vi "RT_BF_LD-400_MFLI_PK_v4.0_measure_voltageR_fourMFLI.vi"() -> ()   [LabVIEW 2016]
uses:
  <instrlib>/Zurich Instruments LabOne/Public/Configure/ziGetValueDemodSampleEx.vi
  <vilib>/Utility/file.llb/Write To Spreadsheet File (DBL).vi
  Labview Drivers/lake_shore_372/Lake Shore 372/Lake Shore 372.lvlib
  <instrlib>/Zurich Instruments LabOne/Zurich Instruments LabOne.lvlib
panel:
  in  "Number average":i32=50
  in  "Current 4 (A)":dbl=1e-09
  in  "Current 3 (A)":dbl=1e-06
  in  "Current 2 (A)":dbl=2e-06
  in  "Current 1 (A)":dbl=2e-06
  in  "MFLI 4 Address":string="DEV3637"
  in  "Device 4 details:":string="VOM133_27.777777Hz_1nA"
  in  "Delay(s) after each data point":dbl format="%#_13g"
  in  "Device 3 details:":string="VOM136_37.7777777Hz_1uA"
  in  "MFLI 3 Address":string="DEV3647"
  in  "MFLI 2 Address":string="DEV4496"
  in  "MFLI 1 Address":string="DEV4382"
  in  "Device 2 details:":string="VOM111_7.919Hz_2uA"
  in  "Device 1 details:":string="VOM134_17.77777Hz_2uA"
  in  "STOP":bool
  out "Device details":string="Device details: \rDevice 1 details: VOM134_17.77777Hz_2uA\tDevice 2 details: VOM111_7.919Hz_2uA\tDevice 3 details: VOM136_37.7777777Hz_1uA\tDevice 4 details: VOM133_27.777777Hz_1nA\t\r"
  out "data":ext[](array[numeric])=[0.0080852, 9923.583, 0.16276936015514457, 1.6064700025522405e-08, 9.869609372556507e-08, 0.27307549143227666, 2.7272832558602143e-08, 9.987286817852663e-08]
  out "path":path=path "D:/Mostafa/17-06-2021/001_RT_cooldown"
  in  "Path":path=path "D:/Mostafa/17-06-2021/001_RT_cooldown"
  in  "Tab Control":enum32{"Page 1", "Page 2"}(tab)
  out "Resistance vs time":cluster{dbl[], dbl[]}[](graph)
  out "Resistance 1 (ohm)":dbl=0.16276936015514457 format="%#_13g"
  out "Voltage 1 (V)":dbl=1.6064700025522405e-08 format="%#_4g"
  out "elapsed time (min)":dbl=165.39305000000002
  out "elapsed time (s)":dbl=9923.583
  out "T MXC (K)":dbl=0.0080852
  out "Resistance vs T":cluster{dbl[], dbl[]}[](graph)
  out "Voltage 2 (V)":dbl=2.7272832558602143e-08 format="%#_4g"
  out "Resistance 2 (ohm)":dbl=0.27307549143227666 format="%#_13g"
  out "Resistance 3 (ohm)":dbl format="%#_13g"
  out "Voltage 3 (V)":dbl=2.7272832558602143e-08 format="%#_4g"
  out "Resistance 4 (ohm)":dbl=0.16276936015514457 format="%#_13g"
  out "Voltage 4 (V)":dbl=2.7272832558602143e-08 format="%#_4g"
  out "Updates":string="- Using shift register to get data from MFLI\n- Using read demod instead of poll function\n- Measuring 2 devices using MFLI at the same time"
  out "Error Out":errorcluster
  # "Use this button to abort the measurement"
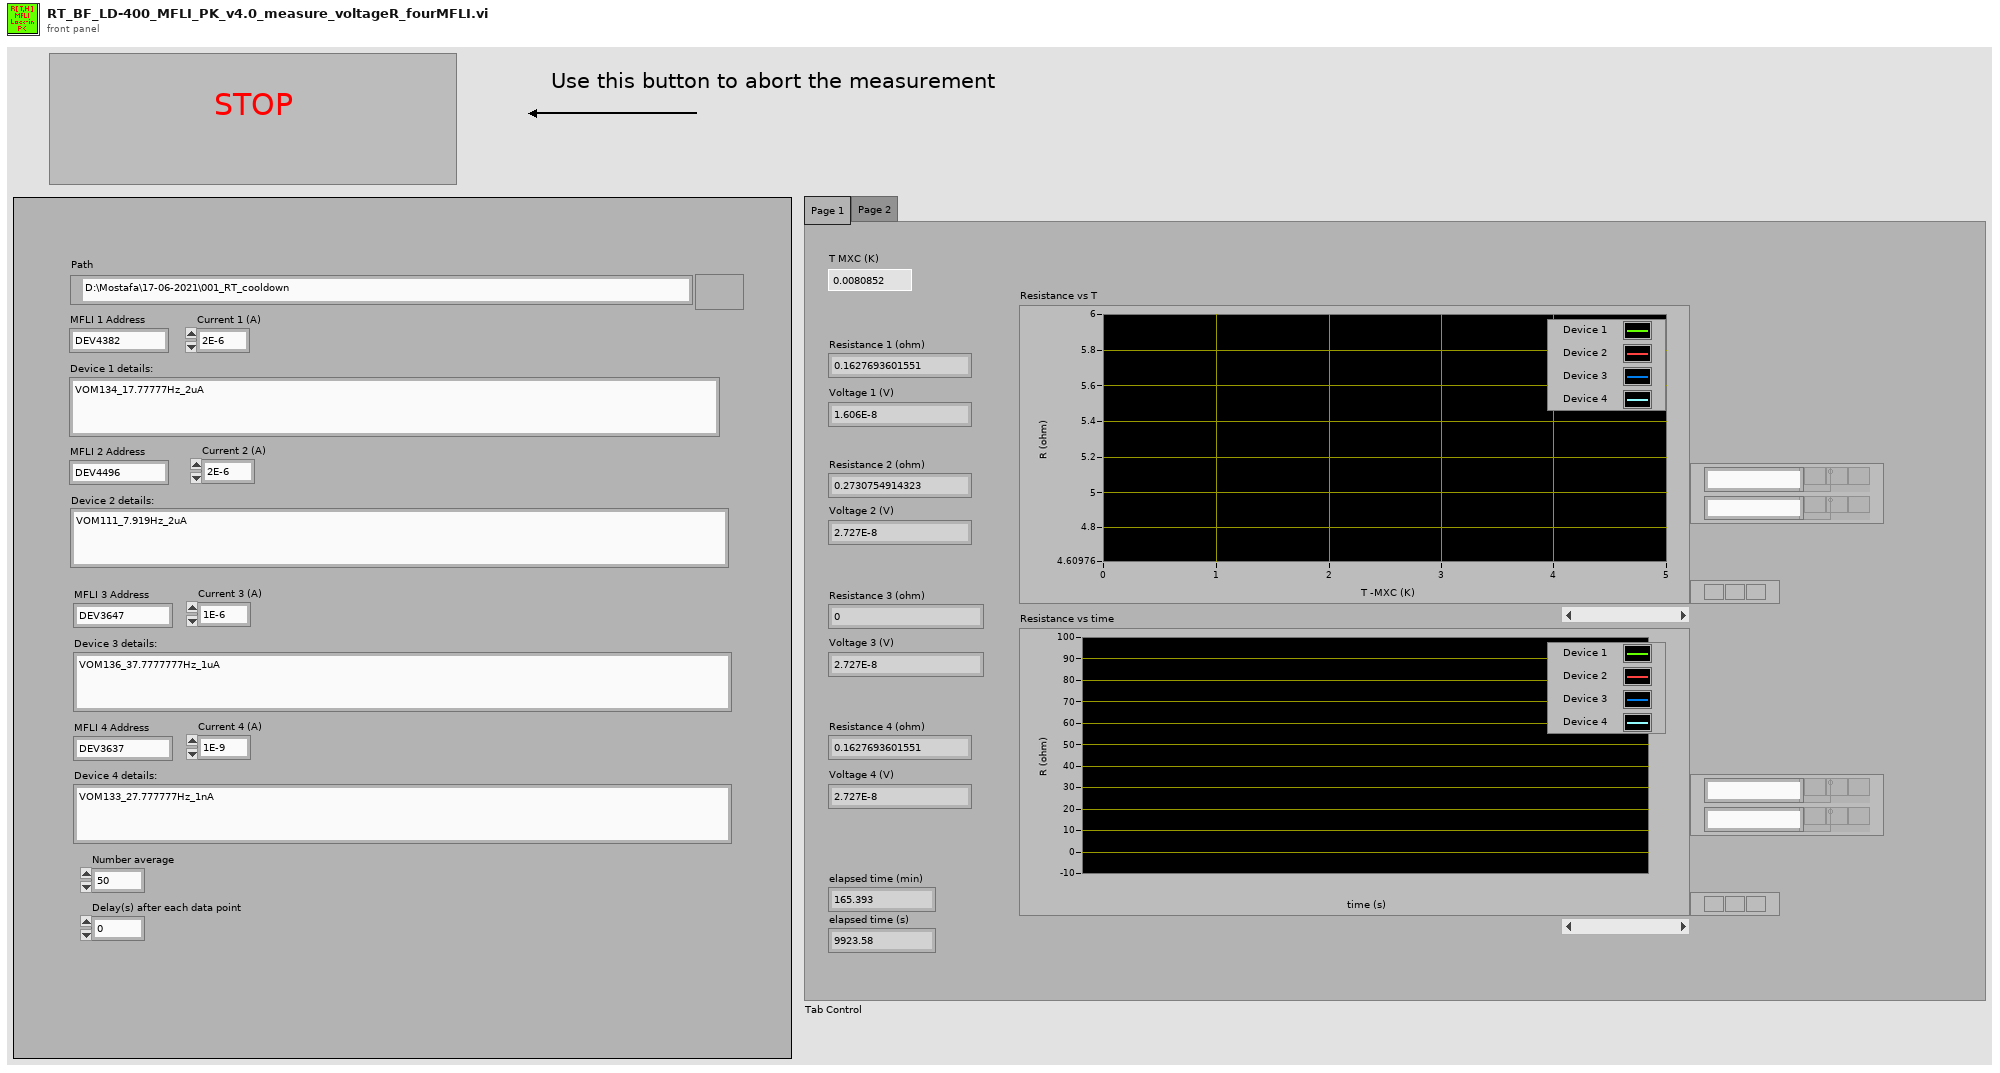
[diagram p1: front panel]
types:
  T1 = enum16{"open", "replace", "create", "open or create", "replace or create", "replace or create with confirmation"}
  T2 = typedef "Zurich Instruments LabOne.lvlib/ziTypeHandle.ctl" = cluster{"handleValid":bool, "Conn":u64, "Path Prefix":string, "Handle":u64, "Connected":bool, "Clockbase(s)":dbl}
  T3 = typedef "Zurich Instruments LabOne.lvlib/ziTypeDemodSampleSingle.ctl" = cluster{"Timestamps (ticks)":u64, "X (Vrms)":dbl, "Y (Vrms)":dbl, "Osc Phase (deg)":dbl, "Freq (Hz)":dbl, "DIO":u32, "AuxIn0 (V)":dbl, "AuxIn1 (V)":dbl, "Trigger":u32}
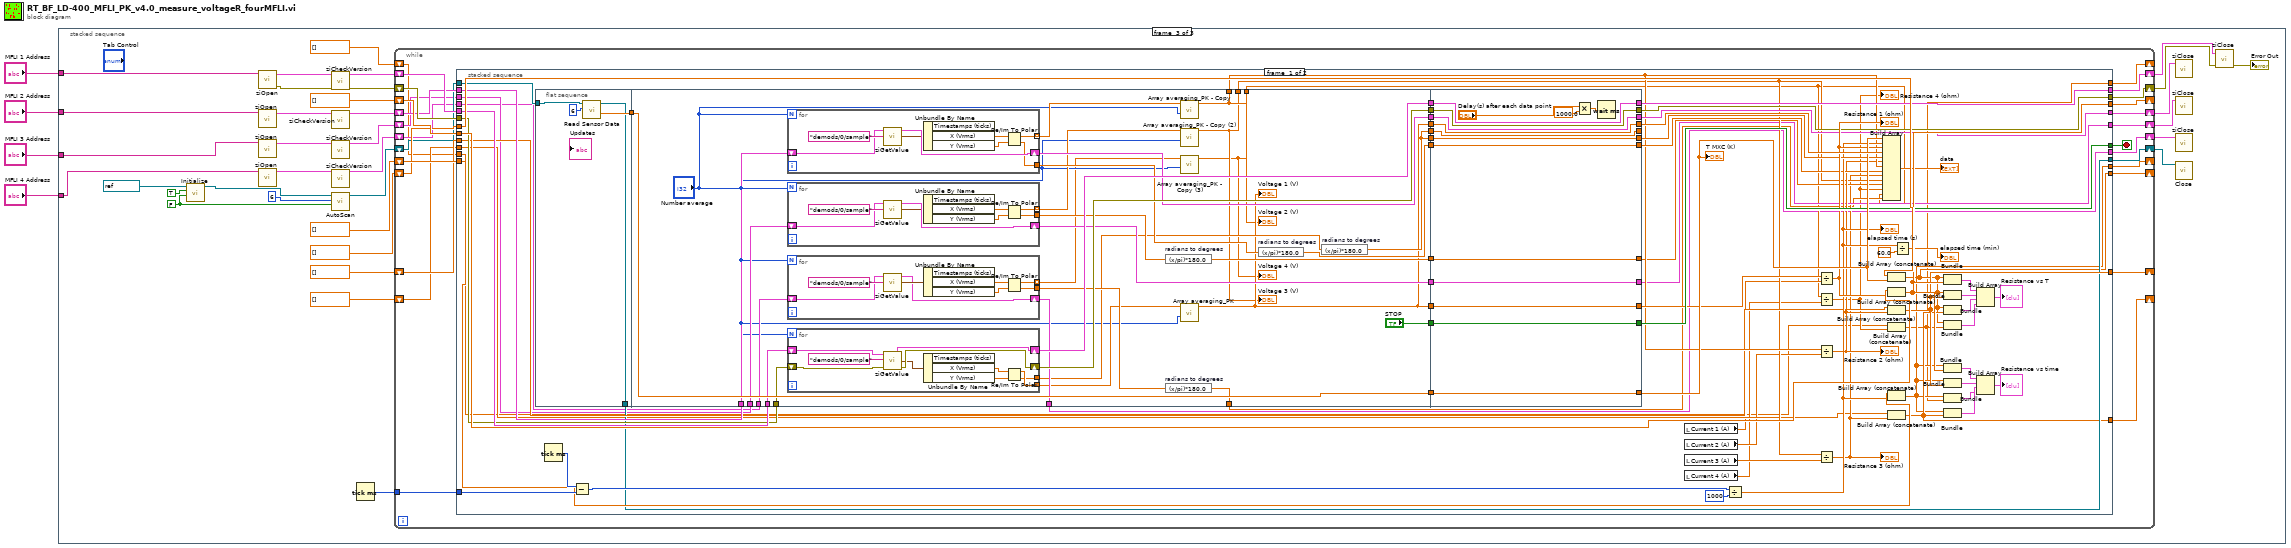
[diagram p0: block diagram]
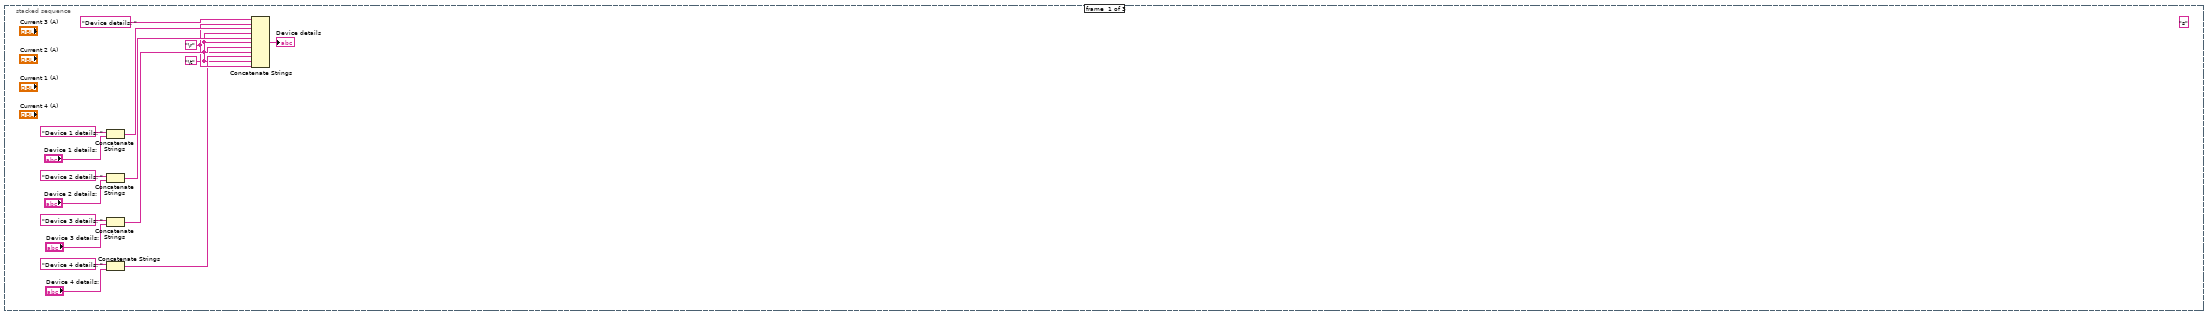
[diagram p2: hidden frame]
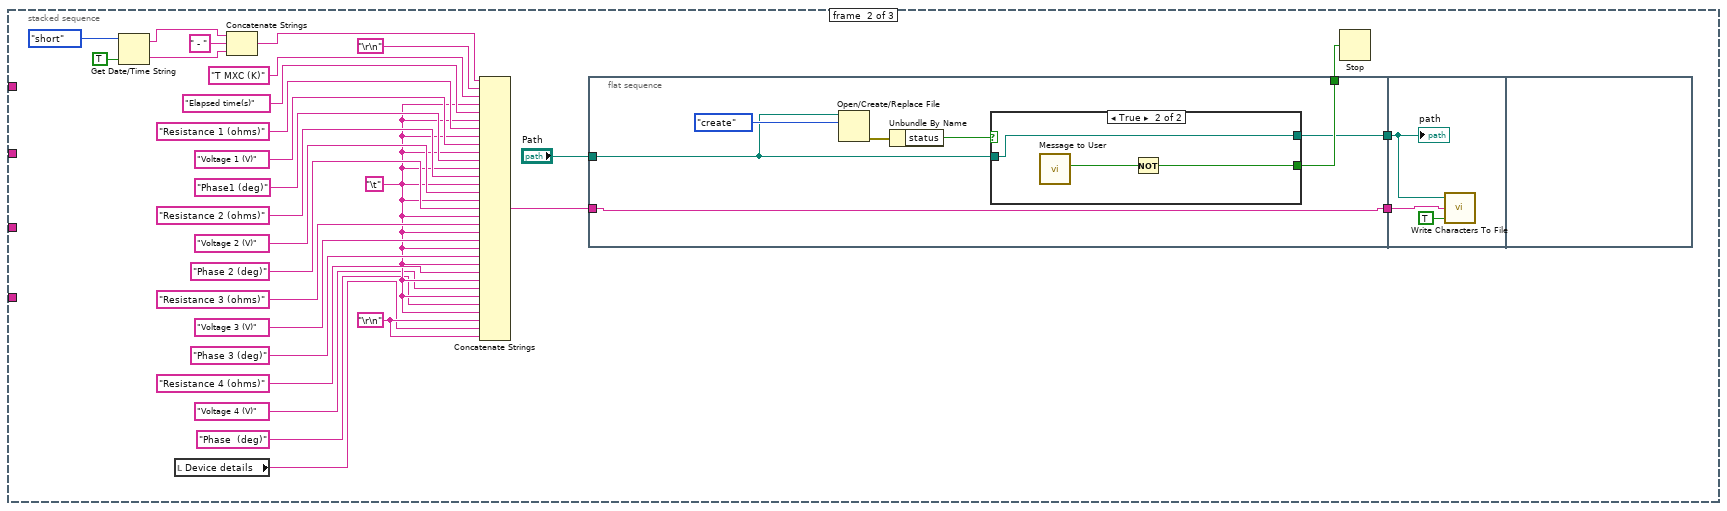
[diagram p3: hidden frame]
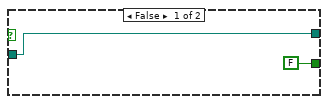
[diagram p4: hidden frame]
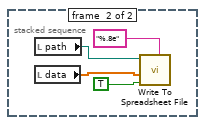
[diagram p5: hidden frame]
diagram:
  n1 = stacked-sequence {
    tunnel: "MFLI 1 Address" -> [_ _ w87]
    tunnel: "MFLI 2 Address" -> [_ _ w85]
    tunnel: "MFLI 3 Address" -> [_ _ w74]
    tunnel: "MFLI 4 Address" -> [_ _ w68]
    frame #0 {
      (unwired) "s"
      w7 = "\r"
      w5 = "\t"
      n2 = Concatenate Strings("Device 1 details: ", "Device 1 details:") -> (w14:string)
      n3 = Concatenate Strings("Device 2 details: ", "Device 2 details:") -> (w13:string)
      n4 = Concatenate Strings("Device 3 details: ", "Device 3 details:") -> (w10:string)
      n5 = Concatenate Strings("Device 4 details: ", "Device 4 details:") -> (w6:string)
      n6 = Concatenate Strings("Device details: ", w7, w14, w5, w13, w5, w10, w5, w6, w5, w7) -> (→"Device details":string)
    }
    frame #1 {
      w26 = "\r\n"
      w23 = "\t"
      n7 = Get Date/Time String(date format (0)=enum16{"short", "long", "abbreviated"}."short", want seconds? (F)=TRUE) -> (date string=w43:string, time string=w42:string)  [unwired: 1 in]
      n8 = local read "Device details"() -> (w25:string)
      n9 = Concatenate Strings(w43, " - " ("string"), w42) -> (w38:string)
      n10 = Concatenate Strings(w38, "\r\n", "T MXC (K)" ("string"), w23, "Elapsed time(s)" ("string"), w23, "Resistance 1 (ohms)" ("string"), w23, "Voltage 1 (V)", w23, "Phase1 (deg)", w23, "Resistance 2 (ohms)" ("string"), w23, "Voltage 2 (V)", w23, "Phase 2 (deg)", w23, "Resistance 3 (ohms)" ("string"), w23, "Voltage 3 (V)", w23, "Phase 3 (deg)", w23, "Resistance 4 (ohms)" ("string"), w23, "Voltage 4 (V)", w23, "Phase  (deg)", w23, w26, w25, w26) -> (w47:string)
      n11 = flat-sequence {
        tunnel: "Path" -> [w50]
        tunnel: w47 -> [w53]
        tunnel: [w53] -> w46
        tunnel: [w52] -> w36
        tunnel: [w51] -> w39
        tunnel: w46 -> [w63]
        tunnel: w39 -> [w62]
        frame #0 {
          n12 = Open/Create/Replace File(file path (use dialog)=w50, operation (0:open)=T1."create") -> (error out=w56:errorcluster)  [unwired: 4 in, 2 out]
          n13 = Unbundle By Name(w56) -> ("status"=w54:bool)
          n14 = case shown="True" w54 {
            tunnel: [FALSE ("Yes") w60] -> w52
            tunnel: [w57 w59] -> w51
            tunnel: w50 -> [w57 w59]
            frame False {
            }
            frame True {
              n15 = call "Message to User"() -> ("Yes"=w61:bool)  [unwired: 10 in, 1 out]
              n16 = Not(x=w61) -> (.not. x?=w60:bool)
            }
          }
        }
        frame #1 {
          n17 = call <vilib>:"Write Characters To File.vi"("append to file? (new file:F)"=TRUE, "character string"=w63, "file path (dialog if empty)"=w62) -> ()  [unwired: 2 in, 1 out]
          "path" <- w62
        }
        frame #2 {
        }
      }
      n18 = Stop(stop? (T)=w36) -> ()
    }
    frame #2 {
      w76 = FALSE
      n19 = call "Initialize.vi"("Reset (True)"=w76, "ID Query (True)"=TRUE, "VISA resource name"=refnum<visa-resource-name> "COM3" ("GPIB Mercury ITC")) -> ("VISA resource name out"=w78:refnum<visa-resource-name>)  [unwired: 7 in, 1 out]
      n20 = call <instrlib>:"ziOpen.vi"("Address"=w87) -> ("Error Out"=w93:errorcluster, "HandleOut"=w94:T2)  [unwired: 3 in, 1 out]
      n21 = call <instrlib>:"ziOpen.vi"("Address"=w85) -> ("HandleOut"=w86:T2)  [unwired: 3 in, 2 out]
      n22 = call <instrlib>:"ziOpen.vi"("Address"=w74) -> ("HandleOut"=w73:T2)  [unwired: 3 in, 2 out]
      n23 = call <instrlib>:"ziOpen.vi"("Address"=w68) -> ("HandleOut"=w69:T2)  [unwired: 3 in, 2 out]
      n24 = call <instrlib>:"ziCheckVersion.vi"("Handle In"=w94, "Error In"=w93) -> ("Handle Out"=w92:T2, "Error Out"=w89:errorcluster)  [unwired: 11 in, 1 out]
      n25 = call <instrlib>:"ziCheckVersion.vi"("Handle In"=w86) -> ("Handle Out"=w83:T2)  [unwired: 12 in, 2 out]
      n26 = call <instrlib>:"ziCheckVersion.vi"("Handle In"=w73) -> ("Handle Out"=w72:T2)  [unwired: 12 in, 2 out]
      n27 = call <instrlib>:"ziCheckVersion.vi"("Handle In"=w69) -> ("Handle Out"=w66:T2)  [unwired: 12 in, 2 out]
      n28 = call "AutoScan.vi"("Autoscan (F: Off)"=w76, "Channel (1:1)"=6, "VISA resource name"=w78) -> ("VISA resource name out"=w75:refnum<visa-resource-name>)  [unwired: 7 in, 1 out]
      n29 = Tick Count (ms)() -> (millisecond timer value=w97:u32)
      n30 = while {
        shift-right: [w119] -> _
        shift-left: dbl[] [] -> [w124]
        tunnel: w97 -> [w123]
        shift-right: [w118] -> _
        shift-left: dbl[] [] -> [w122]
        shift-right: [w120] -> _
        shift-left: dbl[] [] -> [w121]
        shift-right: [w115] -> w91
        shift-left: w92 -> [w117]
        shift-right: [w113] -> w88
        shift-left: w89 -> [w114]
        shift-right: [w112] -> w84
        shift-left: w83 -> [w111]
        shift-right: [w109] -> _
        shift-left: dbl[] [] -> [w110]
        shift-right: [w107] -> w81
        shift-left: w75 -> [w108]
        shift-right: [w105] -> w71
        shift-left: w72 -> [w106]
        shift-right: [w103] -> _
        shift-left: dbl[] [] -> [w104]
        shift-right: [w102] -> w67
        shift-left: w66 -> [w101]
        shift-right: [w99] -> _
        shift-left: dbl[] [] -> [w100]
        stop <- w116 stop-if-true
        n31 = stacked-sequence {
          tunnel: w124 -> [w194 _]
          tunnel: w123 -> [w198 _]
          tunnel: w122 -> [w195 _]
          tunnel: w121 -> [w193 _]
          tunnel: [w127 _] -> w120
          tunnel: [w192 _] -> w119
          tunnel: [w129 _] -> w118
          tunnel: [w185 _] -> w116
          tunnel: w117 -> [w181 _]
          tunnel: [w180 _] -> w115
          tunnel: w114 -> [w179 _]
          tunnel: [w178 _] -> w113
          tunnel: w111 -> [w176 _]
          tunnel: [w175 _] -> w112
          tunnel: w110 -> [w171 _]
          tunnel: [w166 _] -> w109
          tunnel: w108 -> [w162 _]
          tunnel: [w161 _] -> w107
          tunnel: w106 -> [w160 _]
          tunnel: [w157 _] -> w105
          tunnel: w104 -> [w153 _]
          tunnel: [w152 _] -> w103
          tunnel: w101 -> [w133 _]
          tunnel: [w132 _] -> w102
          tunnel: w100 -> [w126 _]
          tunnel: [w125 _] -> w99
          frame #0 {
            n32 = flat-sequence {
              tunnel: w162 -> [w200]
              tunnel: [w201] -> w177
              tunnel: [w199] -> w161
              tunnel: [w210] -> w147
              tunnel: [w231] -> w146
              tunnel: ["STOP"] -> w145
              tunnel: [w210] -> w144
              tunnel: [w229] -> w143
              tunnel: [w229] -> w142
              tunnel: [w228] -> w141
              tunnel: [w227] -> w140
              tunnel: [w226] -> w139
              tunnel: [w225] -> w138
              tunnel: [w224] -> w137
              tunnel: [w223] -> w136
              tunnel: [w203] -> w134
              tunnel: [w221] -> w135
              tunnel: w133 -> [w220]
              tunnel: [w219] -> w132
              tunnel: [w208] -> w172
              tunnel: w176 -> [w216]
              tunnel: w177 -> [w231]
              tunnel: w181 -> [w214]
              tunnel: w179 -> [w213]
              tunnel: w160 -> [w218]
              tunnel: [w206] -> w159
              tunnel: [w269] -> w157
              tunnel: [w270] -> w158
              tunnel: [w271] -> w173
              tunnel: [w272] -> w175
              tunnel: [w273] -> w178
              tunnel: [w274] -> w180
              tunnel: [w275] -> w182
              tunnel: [w276] -> _
              tunnel: [w277] -> w184
              tunnel: [w278] -> w185
              tunnel: [w279] -> w186
              tunnel: [w280] -> w188
              tunnel: w147 -> [w280]
              tunnel: w146 -> [w279]
              tunnel: w145 -> [w278]
              tunnel: w144 -> [w277]
              tunnel: w143 -> [w276]
              tunnel: w142 -> [w275]
              tunnel: w141 -> [w274]
              tunnel: w140 -> [w273]
              tunnel: w139 -> [w272]
              tunnel: w138 -> [w271]
              tunnel: w137 -> [w270]
              tunnel: w136 -> [w269]
              frame #0 {
                n33 = call "Read Sensor Data.vi"("Channel (1:1)"=6, "VISA resource name"=w200) -> ("Kelvin Reading"=w201:dbl, "VISA resource name out"=w199:refnum<visa-resource-name>)  [unwired: 4 in, 4 out]
              }
              frame #1 {
                n34 = for {
                  N: "Number average" -> [_]
                  tunnel: [w243] -> w209 mode=indexing
                  tunnel: [w242] -> w215
                  shift-right: [w249] -> w226
                  shift-left: w216 -> [w247]
                  n35 = call-poly <instrlib>:"ziGetValue.vi"("Path"="demods/0/sample", "Handle In"=w247) -> ("Demod Sample Out"=w246:T3, "Handle Out"=w249:T2)  [unwired: 1 in, 1 out]
                  n36 = Unbundle By Name(w246) -> ("X (Vrms)"=w245:dbl, "Y (Vrms)"=w244:dbl)  [unwired: 1 out]
                  n37 = Re/Im To Polar(2:w244, 3:w245) -> (0:w242:dbl, 1:w243:dbl)
                }
                n38 = for {
                  N: "Number average" -> [_]
                  tunnel: [w259] -> w207 mode=indexing
                  tunnel: [w258] -> w217
                  shift-right: [w265] -> w223
                  shift-left: w218 -> [w260]
                  n39 = call-poly <instrlib>:"ziGetValue.vi"("Path"="demods/0/sample", "Handle In"=w260) -> ("Demod Sample Out"=w263:T3, "Handle Out"=w265:T2)  [unwired: 1 in, 1 out]
                  n40 = Unbundle By Name(w263) -> ("X (Vrms)"=w262:dbl, "Y (Vrms)"=w261:dbl)  [unwired: 1 out]
                  n41 = Re/Im To Polar(2:w261, 3:w262) -> (0:w258:dbl, 1:w259:dbl)
                }
                n42 = for {
                  N: "Number average" -> [_]
                  tunnel: [w253] -> w222
                  tunnel: [w252] -> w204 mode=indexing
                  shift-right: [w250] -> w219
                  shift-left: w220 -> [w251]
                  n43 = call-poly <instrlib>:"ziGetValue.vi"("Path"="demods/0/sample", "Handle In"=w251) -> ("Demod Sample Out"=w254:T3, "Handle Out"=w250:T2)  [unwired: 1 in, 1 out]
                  n44 = Unbundle By Name(w254) -> ("X (Vrms)"=w256:dbl, "Y (Vrms)"=w255:dbl)  [unwired: 1 out]
                  n45 = Re/Im To Polar(2:w255, 3:w256) -> (0:w253:dbl, 1:w252:dbl)
                }
                n46 = for {
                  N: "Number average" -> [_]
                  tunnel: [w241] -> w211 mode=indexing
                  tunnel: [w232] -> w212
                  shift-right: [w240] -> w228
                  shift-left: w214 -> [w236]
                  shift-right: [w239] -> w227
                  shift-left: w213 -> [w235]
                  n47 = call-poly <instrlib>:"ziGetValue.vi"("error in"=w235, "Path"="demods/0/sample", "Handle In"=w236) -> ("error out"=w239:errorcluster, "Demod Sample Out"=w237:T3, "Handle Out"=w240:T2)
                  n48 = Unbundle By Name(w237) -> ("X (Vrms)"=w234:dbl, "Y (Vrms)"=w233:dbl)  [unwired: 1 out]
                  n49 = Re/Im To Polar(2:w233, 3:w234) -> (0:w232:dbl, 1:w241:dbl)
                }
                n50 = expression code="(x/pi)*180.0" "radians to degrees"(w217) -> (w224:dbl)
                n51 = expression code="(x/pi)*180.0" "radians to degrees"(w222) -> (w221:dbl)
                n52 = call "Array averaging_PK - Copy.vi"("Number averaging"="Number average", "numeric array"=w209) -> ("Average value"=w208:dbl)  [unwired: 9 in]
                "Voltage 2 (V)" <- w208
                n53 = call "Array averaging_PK - Copy (2).vi"("Number averaging"="Number average", "numeric array"=w207) -> ("Average value"=w206:dbl)  [unwired: 9 in]
                "Voltage 3 (V)" <- w206
                n54 = call "Array averaging_PK - Copy (3).vi"("Number averaging"="Number average", "numeric array"=w204) -> ("Average value"=w203:dbl)  [unwired: 9 in]
                "Voltage 4 (V)" <- w203
                n55 = call "Array averaging_PK.vi"("Number averaging"="Number average", "numeric array"=w211) -> ("Average value"=w210:dbl)  [unwired: 9 in]
                "Voltage 1 (V)" <- w210
                n56 = expression code="(x/pi)*180.0" "radians to degrees"(w215) -> (w225:dbl)
                n57 = expression code="(x/pi)*180.0" "radians to degrees"(w212) -> (w229:dbl)
              }
              frame #2 {
                n58 = Multiply(x="Delay(s) after each data point", y=1000.0) -> (x*y=w268:dbl)
                n59 = Wait (ms)(milliseconds to wait=w268) -> ()  [unwired: 1 out]
              }
            }
            n60 = Tick Count (ms)() -> (millisecond timer value=w196:u32)
            n61 = Subtract(x=w196, y=w198) -> (x-y=w197:u32)
            n62 = local read "Current 1 (A)"() -> (w151:dbl)
            n63 = local read "Current 2 (A)"() -> (w150:dbl)
            n64 = local read "Current 3 (A)"() -> (w149:dbl)
            n65 = local read "Current 4 (A)"() -> (w148:dbl)
            n66 = Divide(x=w197, y=u32 1000) -> (x/y=w174:dbl)
            "elapsed time (s)" <- w174
            n67 = Divide(x=w184, y=w151) -> (x/y=w183:dbl)
            "Resistance 1 (ohm)" <- w183
            n68 = Divide(x=w134, y=w148) -> (x/y=w130:dbl)
            "Resistance 4 (ohm)" <- w130
            n69 = Divide(x=w172, y=w150) -> (x/y=w170:dbl)
            "Resistance 2 (ohm)" <- w170
            n70 = Divide(x=w159, y=w149) -> (x/y=w156:dbl)
            "Resistance 3 (ohm)" <- w156
            n71 = Build Array(w186, w174, w183, w188, w182, w170, w172, w173, w156, w159, w158, w130, w134, w135) -> (→"data":dbl[])
            n72 = Build Array (concatenate)(w194, w183) -> (w192:dbl[])
            n73 = Build Array (concatenate)(w171, w170) -> (w166:dbl[])
            n74 = Build Array (concatenate)(w126, w130) -> (w125:dbl[])
            n75 = Build Array (concatenate)(w153, w156) -> (w152:dbl[])
            n76 = Build Array (concatenate)(w193, w186) -> (w127:dbl[])
            n77 = Build Array (concatenate)(w195, w174) -> (w129:dbl[])
            n78 = Divide(x=w174, y=60.0) -> (x/y=→"elapsed time (min)":dbl)
            n79 = Bundle(w127, w192) -> (w164:cluster{dbl[], dbl[]})  [unwired: 1 in]
            n80 = Bundle(w127, w166) -> (w165:cluster{dbl[], dbl[]})  [unwired: 1 in]
            n81 = Bundle(w127, w152) -> (w155:cluster{dbl[], dbl[]})  [unwired: 1 in]
            n82 = Bundle(w127, w125) -> (w128:cluster{dbl[], dbl[]})  [unwired: 1 in]
            n83 = Bundle(w129, w192) -> (w169:cluster{dbl[], dbl[]})  [unwired: 1 in]
            n84 = Bundle(w129, w166) -> (w168:cluster{dbl[], dbl[]})  [unwired: 1 in]
            n85 = Bundle(w129, w125) -> (w131:cluster{dbl[], dbl[]})  [unwired: 1 in]
            n86 = Bundle(w129, w152) -> (w154:cluster{dbl[], dbl[]})  [unwired: 1 in]
            n87 = Build Array(w164, w165, w155, w128) -> (→"Resistance vs T":cluster{dbl[], dbl[]}[])
            n88 = Build Array(w169, w168, w154, w131) -> (→"Resistance vs time":cluster{dbl[], dbl[]}[])
            "T MXC (K)" <- w186
          }
          frame #1 {
            n89 = local read "path"() -> (w284:path)
            n90 = local read "data"() -> (w282:ext[])
            n91 = call-poly <vilib>:"Write To Spreadsheet File.vi"("format (%.3f)"="%.8e", "append to file? (new file:F)"=TRUE, "1D data"=w282, "file path (dialog if empty)"=w284) -> ()  [unwired: 4 in, 1 out]
          }
        }
      }
      n92 = call <instrlib>:"ziClose.vi"("Handle In"=w84) -> ()  [unwired: 1 in, 4 out]
      n93 = call <instrlib>:"ziClose.vi"("Handle In"=w71) -> ()  [unwired: 1 in, 4 out]
      n94 = call <instrlib>:"ziClose.vi"("Handle In"=w67) -> ()  [unwired: 1 in, 4 out]
      n95 = call "Close.vi"("VISA resource name"=w81) -> ()  [unwired: 10 in, 1 out]
      n96 = call <instrlib>:"ziClose.vi"("Error In"=w88, "Handle In"=w91) -> ("Error Out"=→"Error Out":errorcluster)  [unwired: 3 out]
    }
  }
